vi "Digital Initialize.vi"(8 "error in (no error)":errorcluster, 11 "Semiconductor Module Context":T1) -> (0 "error out":errorcluster)   [LabVIEW 2014]
uses:
  <vilib>/NI_TestStand_SemiconductorModule/NI_TestStand_Semiconductor_Module.lvlibp/PinMap/General/SemiconductorModuleContext.ctl
  <instrlib>/niDigital/niDigital.llb/niDigital Load Specifications Levels and Timing (Multiple).vi
  <instrlib>/niDigital/niDigital.llb/niDigital Create Capture Waveform (Parallel).vi
  <vilib>/NI_TestStand_SemiconductorModule/NI_TestStand_Semiconductor_Module.lvlibp
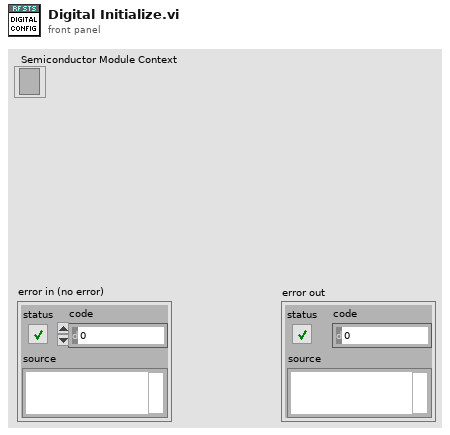
[diagram p1: front panel]
types:
  T1 = typedef "NI_TestStand_Semiconductor_Module.lvlibp/SemiconductorModuleContext.ctl" = refnum<k7>
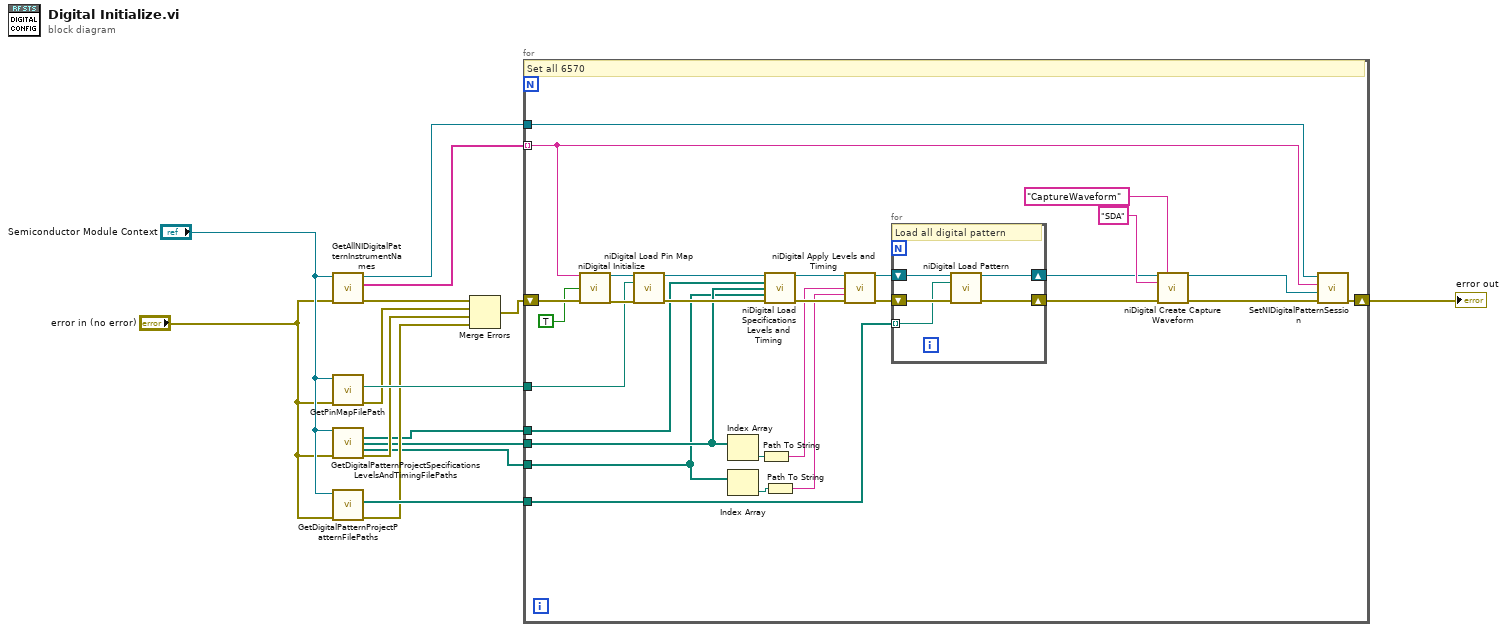
[diagram p0: block diagram]
diagram:
  n1 = call <vilib>:"GetAllNIDigitalPatternInstrumentNames.vi"("error in (no error)"="error in (no error)", "Semiconductor Module Context"="Semiconductor Module Context") -> ("error out"=w12:errorcluster, "Instrument Names"=w15:string[], "Semiconductor Module Context Out"=w14:T1)  [unwired: 7 in]
  n2 = call <vilib>:"GetPinMapFilePath.vi"("error in (no error)"="error in (no error)", "Semiconductor Module Context"="Semiconductor Module Context") -> ("error out"=w11:errorcluster, "Pin Map File Path"=w13:path)  [unwired: 7 in, 1 out]
  n3 = call <vilib>:"GetDigitalPatternProjectSpecificationsLevelsAndTimingFilePaths.vi"("Semiconductor Module Context"="Semiconductor Module Context", "error in (no error)"="error in (no error)") -> ("Specifications File Paths"=w5:path[], "Levels File Paths"=w6:path[], "Timing File Paths"=w4:path[], "error out"=w9:errorcluster)  [unwired: 9 in, 1 out]
  n4 = call <vilib>:"GetDigitalPatternProjectPatternFilePaths.vi"("error in (no error)"="error in (no error)", "Semiconductor Module Context"="Semiconductor Module Context") -> ("error out"=w7:errorcluster, "Pattern File Paths"=w8:path[])  [unwired: 7 in, 1 out]
  n5 = Merge Errors(w12, w11, w9, w7) -> (w10:errorcluster)
  n6 = for {
    shift-right: [w40] -> w3
    shift-left: w10 -> [w43]
    tunnel: w15 -> [w27] mode=indexing
    tunnel: w5 -> [w30]
    tunnel: w4 -> [w24]
    tunnel: w13 -> [w39]
    tunnel: w14 -> [w37]
    tunnel: w8 -> [w28]
    tunnel: w6 -> [w26]
    # "Set all 6570"
    n7 = call <instrlib>:"niDigital Initialize.vi"("resource name"=w27, "reset (T)"=TRUE ("reset"), "error in"=w43) -> ("instrument handle"=w41:refnum<k15>, "error out"=w42:errorcluster)  [unwired: 11 in]
    n8 = call <instrlib>:"niDigital Load Pin Map.vi"("instrument handle"=w41, "pin map file"=w39, "error in"=w42) -> ("instrument handle out"=w32:refnum<k15>, "error out"=w36:errorcluster)  [unwired: 11 in]
    n9 = Index Array(array=w26) -> (element=w25:path)  [unwired: 1 in]
    n10 = Index Array(array=w24) -> (element=w23:path)  [unwired: 1 in]
    n11 = Path To String(path=w25) -> (string=w29:string)
    n12 = call-poly <instrlib>:"niDigital Load Specifications Levels and Timing.vi"("instrument handle"=w32, "specifications file paths"=w30, "levels file paths"=w26, "timing file paths"=w24, "error in"=w36) -> ("instrument handle out"=w31:refnum<k15>, "error out"=w35:errorcluster)  [unwired: 9 in]
    n13 = Path To String(path=w23) -> (string=w22:string)
    n14 = call <instrlib>:"niDigital Apply Levels and Timing.vi"("instrument handle"=w31, "levels sheet"=w29, "timing sheet"=w22, "error in"=w35) -> ("instrument handle out"=w33:refnum<k15>, "error out"=w34:errorcluster)  [unwired: 10 in]
    n15 = for {
      shift-right: [w45] -> w19
      shift-left: w33 -> [w48]
      shift-right: [w46] -> w18
      shift-left: w34 -> [w47]
      tunnel: w28 -> [w44] mode=indexing
      # "Load all digital pattern"
      n16 = call <instrlib>:"niDigital Load Pattern.vi"("instrument handle"=w48, "pattern file"=w44, "error in"=w47) -> ("instrument handle out"=w45:refnum<k15>, "error out"=w46:errorcluster)  [unwired: 11 in]
    }
    n17 = call-poly <instrlib>:"niDigital Create Capture Waveform.vi"("instrument handle"=w19, "waveform name"="CaptureWaveform", "pin list"="SDA" ("waveform name"), "error in"=w18) -> ("instrument handle out"=w17:refnum<k15>, "error out"=w16:errorcluster)  [unwired: 10 in]
    n18 = call <vilib>:"SetNIDigitalPatternSession.vi"("error in (no error)"=w16, "Instrument Session"=w17, "Instrument Name"=w27, "Semiconductor Module Context"=w37) -> ("error out"=w40:errorcluster)  [unwired: 6 in, 1 out]
  }
  "error out" <- w3
